vi "题目1.vi"() -> ()   [LabVIEW 2017]
panel:
  in  "滑钮2":dbl(slide) scale=0.0..10.0
  out "波形图表 2":dbl[](graph)
  in  "滑钮":dbl(slide) scale=0.0..10.0
  out "波形图表":dbl(graph)
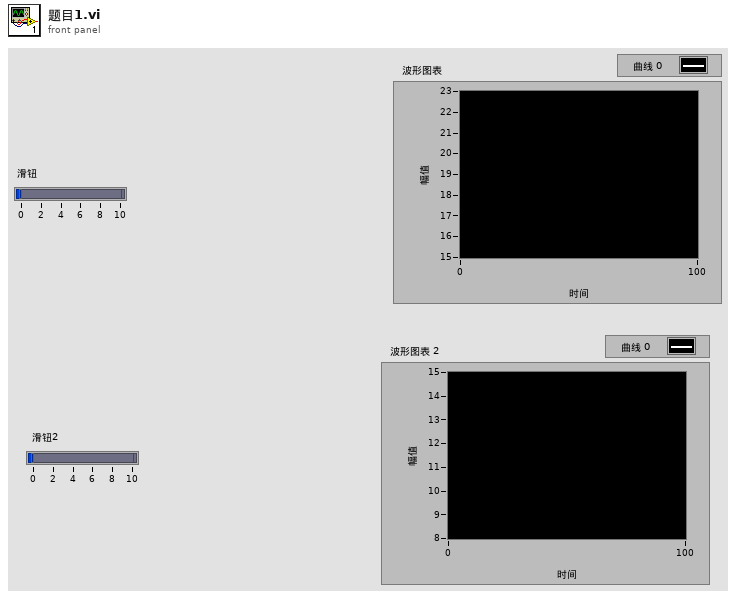
[diagram p1: front panel]
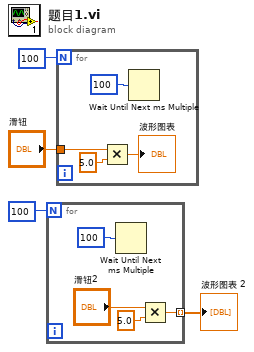
[diagram p0: block diagram]
diagram:
  n1 = for {
    N: 100 -> [_]
    tunnel: [w5] -> w1 mode=indexing
    n2 = Wait Until Next ms Multiple(millisecond multiple=u32 100 ("毫秒倍数")) -> ()  [unwired: 1 out]
    n3 = Multiply(x="滑钮2", y=5.0) -> (x*y=w5:dbl)
  }
  "波形图表 2" <- w1
  n4 = for {
    N: 100 -> [_]
    tunnel: "滑钮" -> [w11]
    n5 = Multiply(x=w11, y=5.0) -> (x*y=→"波形图表":dbl)
    n6 = Wait Until Next ms Multiple(millisecond multiple=100) -> ()  [unwired: 1 out]
  }
